vi "Send Coil Calib to FPGA.vi"(8 "error in (no error)":errorcluster, 11 "Refnum in":T1) -> (0 "error out":errorcluster, 2 "Magnet Configuration Data":T2 {"Coil D Coefficients" format="%_6g"; "Coil C Coefficients" format="%_6g"; "Coil B Coefficients" format="%_6g"; "Scale Factors" format="%_6g"; "Offsets" format="%_6g"; "Temp Coef" format="%_6g"; "Max Coil Temp" format="%_6g"; "Max Coil Volt Dev" format="%_6g"; "Max Coil Currents" format="%_6g"; "Coil Inductances" format="%_6g"; "Pressure Range" format="%_6g"; "Coil A Coefficients" format="%_6g"}, 3 "Refnum out":T1)   [LabVIEW 2020]
doc: "Author: Scott Hannahs <sth@magnet.fsu.edu>\nCopyright 2018 Florida State University, All rights reserved."
uses:
  <vilib>/rvi/interface/nirviReadWriteControl/nirviReadWriteControl.xnode
  FPGA Magnet Config.ctl
  RT Controls/FPGA SCH Digitizer Ref.ctl
  SCH Data Controls/SCH Data 2 RT.ctl
  NiFpgaLv.dll
  <vilib>/Utility/error.llb/Error Cluster From Error Code.vi
  <vilib>/rvi/interface/Simulation/niFpgaSimulationCallBeginRW.vi
  <vilib>/rvi/errors/niLvFpgaAdjustHostInterfaceError.vi
panel:
  # "mH"
  # "kA"
  # "V"
  # "mOhm"
  # "mOhm"
  # "mOhm"
  # "mOhm"
  # "Deg C"
  # "bar"
  # "1/Deg C"
  # "Tin"
  # "Tout"
  # "Pin"
  # "Pout"
  # "I"
  # "WDTin"
  # "PSEnb"
  # "CellFLT"
  # "WDTout"
  # "BTFlt"
  # "BTvolt"
  # "Va"
  # "Vb"
  # "Vc"
  # "Vd"
  # "Tin"
  # "Tout"
  # "Pin"
  # "Pout"
  # "I"
  # "WDTin"
  # "PSEnb"
  # "CellFLT"
  # "WDTout"
  # "BTFlt"
  # "BTvolt"
  # "Va"
  # "Vb"
  # "Vc"
  # "Vd"
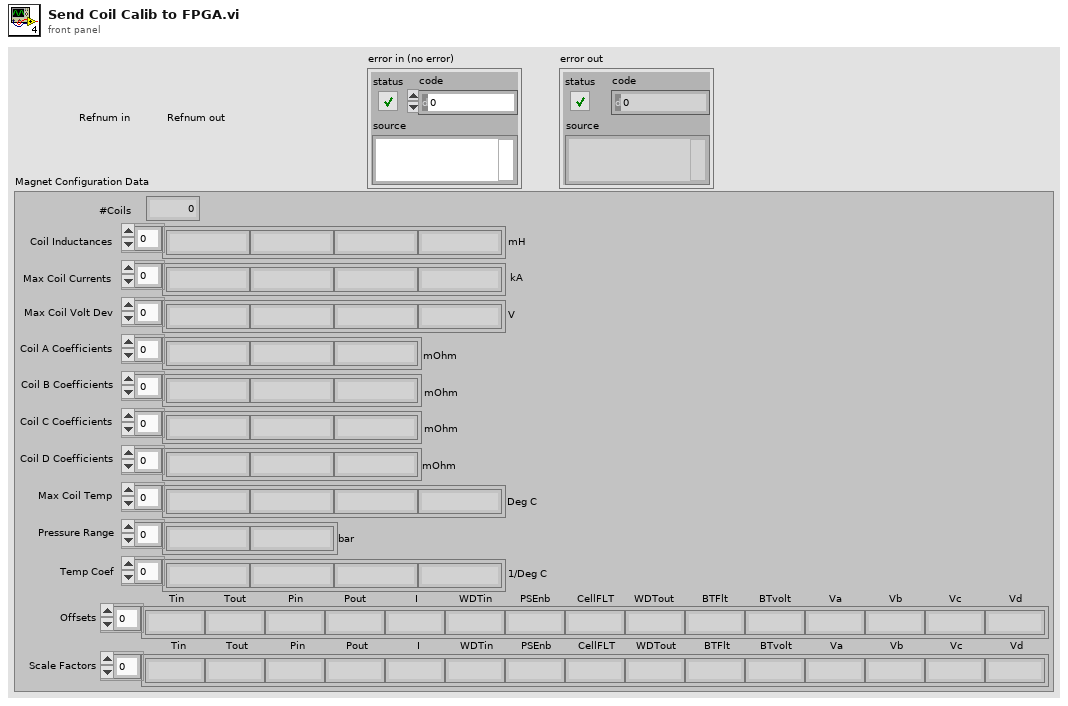
[diagram p1: front panel]
types:
  T1 = typedef "FPGA SCH Digitizer Ref.ctl" = refnum<k20>
  T2 = typedef "FPGA Magnet Config.ctl" = cluster{"#Coils":u32, "Coil Inductances":T3[], "Max Coil Currents":T3[], "Max Coil Volt Dev":T3[], "Coil A Coefficients":T3[], "Coil B Coefficients":T3[], "Coil C Coefficients":T3[], "Coil D Coefficients":T3[], "Max Coil Temp":T3[], " Pressure Range":T3[], "Temp Coef":T3[], "Offsets":T3[], "Scale Factors":T3[]}
  T3 = typedef "SCH Data 2 RT.ctl" = fxp<+/-,38,12>
  T4 = typedef "RMPS Magnet Config.ctl" = cluster{"#Coils":u32, "Coil Inductances":dbl[], "Maximum Coil Currents":dbl[], "Maximum Coil Voltage Deviation":dbl[], "Coil Coefficients":dbl[][], "Maximum Coil Temperatures":dbl[], " Pressure Range":dbl[], "Temp Coef":dbl[], "Offsets":dbl[], "Scale Factors":dbl[], "Cell Name":string}
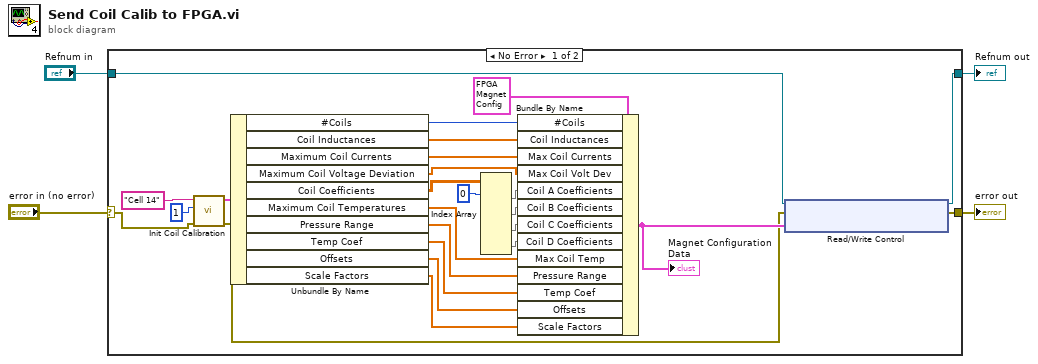
[diagram p0: block diagram]
diagram:
  n1 = case shown="No Error" "error in (no error)" {
    selector: "error in (no error)" -> [w6 w30]
    tunnel: "Refnum in" -> [w9 w31]
    tunnel: [w8 w31] -> w2
    tunnel: [w7 w30] -> w1
    frame No Error {
      n2 = call "Init Coil Calibration.vi"("Magnet ID"="Cell 14", "# Power Supplies"=u32 1, "error in"=w6) -> ("Magnet Configuration Data"=w17:T4, "error out"=w5:errorcluster)  [unwired: 1 in, 4 out]
      n3 = Unbundle By Name(w17) -> ("#Coils"=w13:u32, "Coil Inductances"=w14:dbl[], "Maximum Coil Currents"=w15:dbl[], "Maximum Coil Voltage Deviation"=w16:dbl[], "Coil Coefficients"=w11:dbl[][], "Maximum Coil Temperatures"=w25:dbl[], "Pressure Range"=w26:dbl[], "Temp Coef"=w27:dbl[], "Offsets"=w28:dbl[], "Scale Factors"=w29:dbl[])
      n4 = Index Array(array=w11, index (row) #1=0 ("index (row)")) -> (element #1=w12:dbl[], element #2=w22:dbl[], element #3=w23:dbl[], element #4=w24:dbl[])  [unwired: 7 in]
      n5 = Bundle By Name(cluster=T2 {"#Coils"=0, "Coil Inductances"=[0.0, 0.0, 0.0, 0.0], "Max Coil Currents"=[0.0, 0.0, 0.0, 0.0], "Max Coil Volt Dev"=[0.0, 0.0, 0.0, 0.0], "Coil A Coefficients"=[0.0, 0.0, 0.0], "Coil B Coefficients"=[0.0, 0.0, 0.0], "Coil C Coefficients"=[0.0, 0.0, 0.0], "Coil D Coefficients"=[0.0, 0.0, 0.0], "Max Coil Temp"=[0.0, 0.0, 0.0, 0.0], " Pressure Range"=[0.0, 0.0], "Temp Coef"=[0.0, 0.0, 0.0, 0.0], "Offsets"=[0.0, 0.0, 0.0, 0.0, 0.0, 0.0, 0.0, 0.0, 0.0, 0.0, 0.0, 0.0, 0.0, 0.0, 0.0], "Scale Factors"=[0.0, 0.0, 0.0, 0.0, 0.0, 0.0, 0.0, 0.0, 0.0, 0.0, 0.0, 0.0, 0.0, 0.0, 0.0]} ("Magnet Configuration Data"), "#Coils"=w13, "Coil Inductances"=w14, "Max Coil Currents"=w15, "Max Coil Volt Dev"=w16, "Coil A Coefficients"=w12, "Coil B Coefficients"=w22, "Coil C Coefficients"=w23, "Coil D Coefficients"=w24, "Max Coil Temp"=w25, "Pressure Range"=w26, "Temp Coef"=w27, "Offsets"=w28, "Scale Factors"=w29) -> (w20:T2)
      "Magnet Configuration Data" <- w20
      n6 = xnode "Read/Write Control"("FPGA VI Reference In"=w9, "error in"=w5, "Magnet Configuration Data"=w20) -> ("FPGA VI Reference Out"=w8:T1, "error out"=w7:errorcluster)
    }
    frame Error {
    }
  }
  "Refnum out" <- w2
  "error out" <- w1
